vi "ReadCurrentSettings.vi"(5 "UT340 Simple Controls":refnum<vi>, 7 "UT340 Controls":refnum<vi>, 8 "error in (no error)":errorcluster, 11 "VISA Refnum in":refnum<visa-resource-name>) -> (0 "error out":errorcluster, 1 "UT340 Controls":T1={"High Pass On"=FALSE, "High Pass Filter (MHz)"=1, "Low Pass On"=FALSE, "Low Pass Filter (MHz)"=20, "PE Gain (dB)"=1, "Voltage"=100, "Pulse Width (ns)"=2.0, "Mode"=FALSE, "PC Gain (dB)"=1, "Trig Source"=FALSE, "Rep Rate (Hz)"=0, "PULSE"=FALSE} {"Low Pass Filter (MHz)" min=20 step=1; "High Pass Filter (MHz)" min=1 max=20 step=1; "Pulse Width (ns)" min=2.0 max=71.75; "Voltage" min=100 max=250 step=2; "PC Gain (dB)" min=-6 max=60 step=1; "PE Gain (dB)" min=-6 max=60 step=1}, 3 "VISA Refnum out":refnum<visa-resource-name>)   [LabVIEW 2022 SP3]
uses:
  Controls/UTEX Controls.ctl
  Controls/UTEX Controls Simple.ctl
  PulserGlobals.vi
panel:
  out "error out 2":errorcluster
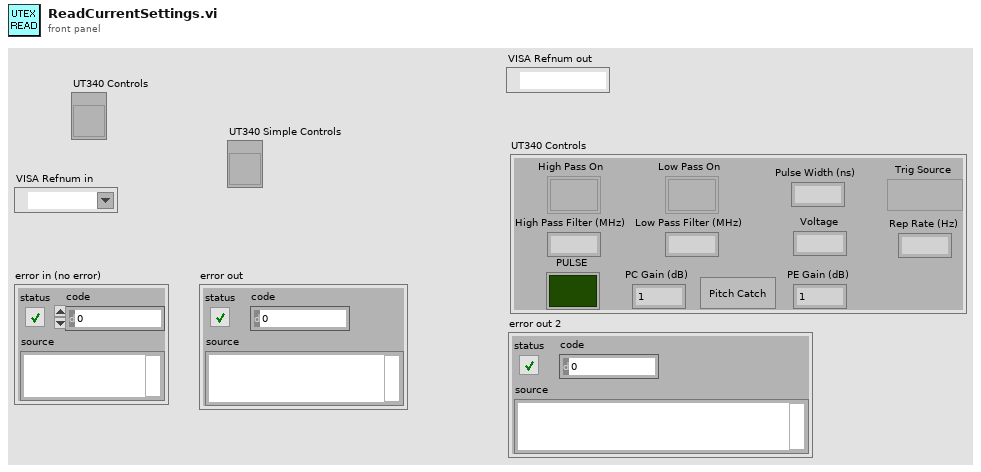
[diagram p1: front panel]
types:
  T1 = typedef "UTEX Controls.ctl" = cluster{"High Pass On":bool, "High Pass Filter (MHz)":i16, "Low Pass On":bool, "Low Pass Filter (MHz)":i16, "PE Gain (dB)":i16, "Voltage":i16, "Pulse Width (ns)":dbl, "Mode":bool, "PC Gain (dB)":i16, "Trig Source":bool, "Rep Rate (Hz)":i16, "PULSE":bool}
  T2 = typedef "UTEX Controls Simple.ctl" = cluster{"PE Gain (dB)":i16, "Voltage":i16}
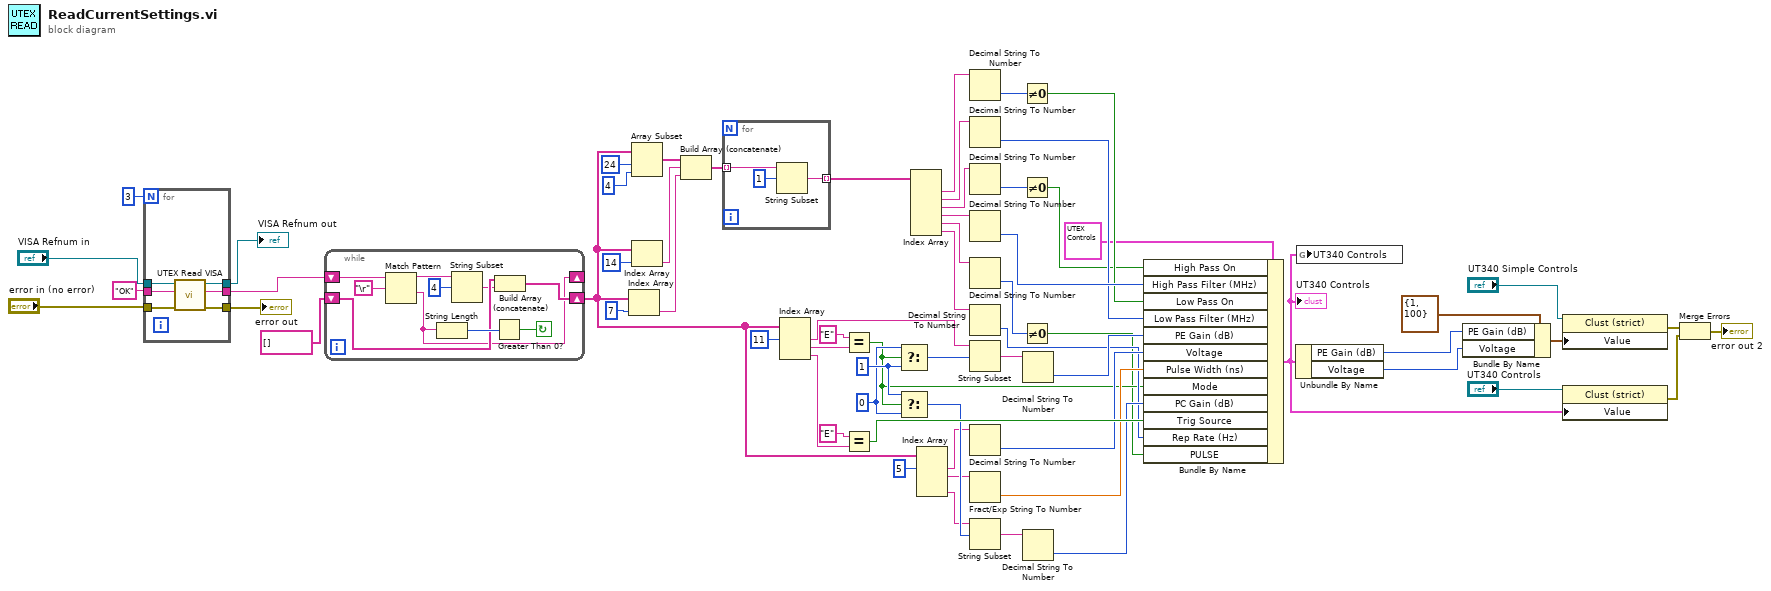
[diagram p0: block diagram]
diagram:
  w46 = 0 ("t")
  w47 = 1 ("offset (0)")
  n1 = for {
    N: 3 -> [_]
    tunnel: "VISA Refnum in" -> [w72]
    tunnel: [w67] -> w2
    tunnel: "OK" ("write buffer") -> [w69]
    tunnel: [w70] -> w17
    tunnel: "error in (no error)" -> [w68]
    tunnel: [w71] -> w18
    n2 = call "UTEX Read VISA.vi"("error in"=w68, "write buffer"=w69, "VISA Refnum in"=w72) -> ("error out"=w71:errorcluster, "read buffer"=w70:string, "VISA Refnum out"=w67:refnum<visa-resource-name>)  [unwired: 6 in]
  }
  "error out" <- w18
  "VISA Refnum out" <- w2
  n3 = while {
    shift-right: [w76] -> _
    shift-left: w17 -> [w79]
    shift-right: [w77] -> w26
    shift-left: string[] [] -> [w80]
    stop <- w81 continue-if-true
    n4 = Match Pattern(string=w79, regular expression="\r") -> (before substring=w74:string, after substring=w76:string)  [unwired: 1 in, 2 out]
    n5 = String Length(string=w76) -> (length=w82:i32)
    n6 = String Subset(string=w74, offset (0)=4) -> (substring=w73:string)  [unwired: 1 in]
    n7 = Greater Than 0?(x=w82) -> (x > 0?=w81:bool)
    n8 = Build Array (concatenate)(w80, w73) -> (w77:string[])
  }
  n9 = Index Array(array=w26, index=7) -> (element=w28:string)
  n10 = Array Subset(array=w26, index=24, length=4) -> (w30:string[])
  n11 = Index Array(array=w26, index=14) -> (element=w31:string)
  n12 = Build Array (concatenate)(w30, w31, w28) -> (w35:string[])
  n13 = for {
    tunnel: w35 -> [w84] mode=indexing
    tunnel: [w83] -> w36 mode=indexing
    n14 = String Subset(string=w84, offset (0)=1) -> (substring=w83:string)  [unwired: 1 in]
  }
  n15 = Index Array(array=w26, index #1=11 ("index")) -> (element #1=w22:string, element #2=w21:string, element #3=w20:string)  [unwired: 2 in]
  n16 = Equal?(x="E", y=w21) -> (x = y?=w45:bool)
  n17 = Equal?(x="E", y=w20) -> (x = y?=w58:bool)
  n18 = Select(t=w46, s=w45, f=w47) -> (s? t:f=w49:i32)
  n19 = Select(t=w47, s=w45, f=w46) -> (s? t:f=w48:i32)
  n20 = Index Array(array=w36) -> (element #1=w60:string, element #2=w38:string, element #3=w64:string, element #4=w63:string, element #5=w34:string, element #6=w27:string)  [unwired: 6 in]
  n21 = Index Array(array=w26, index #1=5 ("index")) -> (element #1=w24:string, element #2=w23:string, element #4=w8:string)  [unwired: 3 in, 1 out]
  n22 = Decimal String To Number(string=w60) -> (number=w42:i32)  [unwired: 2 in, 1 out]
  n23 = Decimal String To Number(string=w38) -> (number=w61:i32)  [unwired: 2 in, 1 out]
  n24 = Decimal String To Number(string=w64) -> (number=w40:i32)  [unwired: 2 in, 1 out]
  n25 = Decimal String To Number(string=w63) -> (number=w62:i32)  [unwired: 2 in, 1 out]
  n26 = Decimal String To Number(string=w34) -> (number=w44:i32)  [unwired: 2 in, 1 out]
  n27 = Decimal String To Number(string=w27) -> (number=w50:i32)  [unwired: 2 in, 1 out]
  n28 = String Subset(string=w22, offset (0)=w49) -> (substring=w52:string)  [unwired: 1 in]
  n29 = Decimal String To Number(string=w24) -> (number=w55:i32)  [unwired: 2 in, 1 out]
  n30 = Fract/Exp String To Number(string=w23) -> (number=w56:dbl)  [unwired: 3 in, 1 out]
  n31 = String Subset(string=w8, offset (0)=w48) -> (substring=w54:string)  [unwired: 1 in]
  n32 = Not Equal To 0?(x=w42) -> (x != 0?=w41:bool)
  n33 = Not Equal To 0?(x=w40) -> (x != 0?=w39:bool)
  n34 = Not Equal To 0?(x=w44) -> (x != 0?=w43:bool)
  n35 = Decimal String To Number(string=w52) -> (number=w51:i32)  [unwired: 2 in, 1 out]
  n36 = Decimal String To Number(string=w54) -> (number=w53:i32)  [unwired: 2 in, 1 out]
  n37 = Bundle By Name(cluster=T1 {"High Pass On"=TRUE, "High Pass Filter (MHz)"=13, "Low Pass On"=FALSE, "Low Pass Filter (MHz)"=85, "PE Gain (dB)"=30, "Voltage"=100, "Pulse Width (ns)"=7.2, "Mode"=TRUE, "PC Gain (dB)"=0, "Trig Source"=TRUE, "Rep Rate (Hz)"=700, "PULSE"=FALSE} ("UT340 Controls"), "High Pass On"=w39, "High Pass Filter (MHz)"=w62, "Low Pass On"=w41, "Low Pass Filter (MHz)"=w61, "PE Gain (dB)"=w51, "Voltage"=w55, "Pulse Width (ns)"=w56, "Mode"=w45, "PC Gain (dB)"=w53, "Trig Source"=w58, "Rep Rate (Hz)"=w50, "PULSE"=w43) -> (w7:T1)
  "UT340 Controls" <- w7
  n38 = Unbundle By Name(w7) -> ("PE Gain (dB)"=w11:i16, "Voltage"=w10:i16)
  n39 = global write "PulserGlobals.vi" "UT340 Controls"(w7) -> ()
  n40 = Bundle By Name(cluster=T2 {"PE Gain (dB)"=1, "Voltage"=100} ("UT340 Controls"), "PE Gain (dB)"=w11, "Voltage"=w10) -> (w12:T2)
  n41 = property class="Clust (strict)"(reference="UT340 Simple Controls", "Value"=w12) -> (error out=w5:errorcluster)  [unwired: 1 in, 1 out]
  n42 = property class="Clust (strict)"(reference="UT340 Controls", "Value"=w7) -> (error out=w3:errorcluster)  [unwired: 1 in, 1 out]
  n43 = Merge Errors(w5, w3) -> (→"error out 2":errorcluster)
